vi "Resize Value Columns.vi"(8 "error in":errorcluster, 9 "Item Names":string[][](array[string]), 10 "Column Header":string[](array[string]), 11 "Report Viewer in":refnum<class "Report Viewer.lvclass">) -> (0 "error out":errorcluster, 3 "Report Viewer out":refnum<class "Report Viewer.lvclass">)   [LabVIEW 2023, in "Report Viewer.lvlib" / "Report Viewer.lvclass"]
uses:
  Library/Report Viewer.lvclass
  Library/Report Viewer.lvclass/Report Viewer.ctl
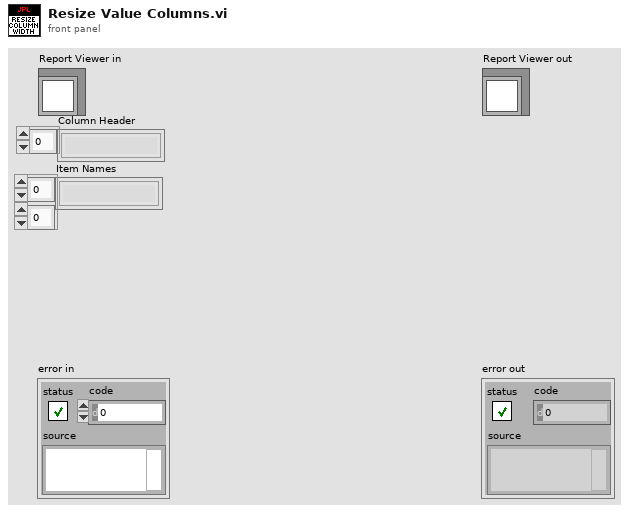
[diagram p1: front panel]
types:
  T1 = enum16{"User-specified Font", "Application Font", "System Font", "Dialog Font"}
  T2 = cluster{"left":i16, "top":i16, "right":i16, "bottom":i16}
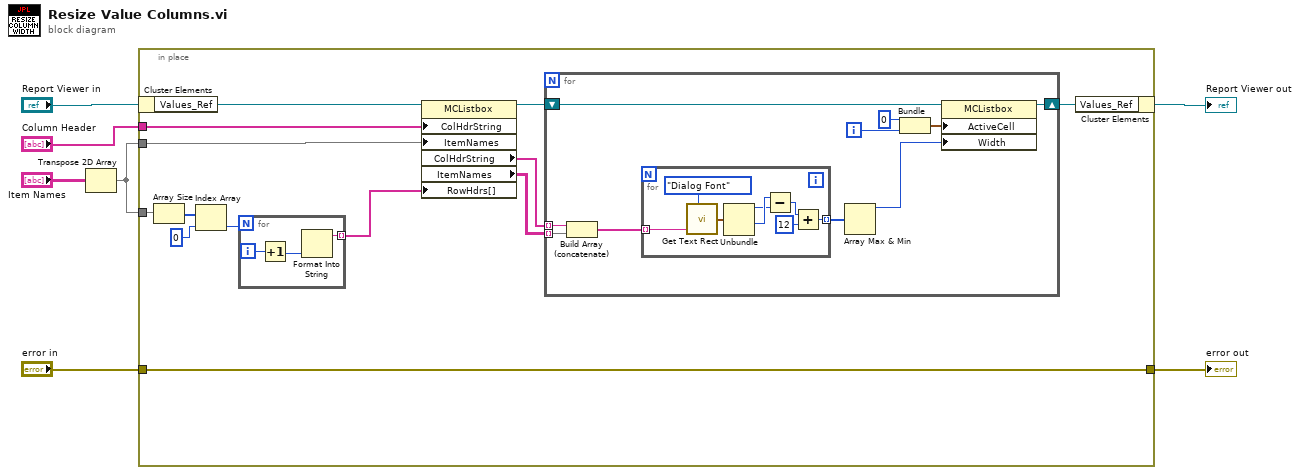
[diagram p0: block diagram]
diagram:
  n1 = Transpose 2D Array(2D array="Item Names") -> (transposed array=w1:string[][])
  n2 = in-place {
    in-place-border: "error in" -> [w15]
    in-place-border: [w15] -> w4
    in-place-border: "Column Header" -> [w14]
    in-place-border: w1 -> [w13]
    in-place-border: w1 -> [w12]
    n3 = in-place-cluster #1("Report Viewer in") -> ("Values_Ref"=w20:refnum<vi>)
    n4 = Array Size(array=w12) -> (size(s)=w11:i32[])
    n5 = Index Array(array=w11, index=0) -> (element=w9:i32)
    n6 = for {
      N: w9 -> [_]
      tunnel: [w21] -> w8 mode=indexing
      i -> [w23]
      n7 = Increment(x=w23) -> (x+1=w22:i32)
      n8 = Format Into String(w22) -> (resulting string=w21:string)  [unwired: 3 in, 1 out]
    }
    n9 = property class="MCListbox"(reference=w20, "ColHdrString"=w14, "ItemNames"=w13, "RowHdrs[]"=w8) -> (reference out=w19:refnum<vi>, "ColHdrString"=w18:string[], "ItemNames"=w17:string[][])  [unwired: 1 in, 1 out]
    n10 = for {
      tunnel: w17 -> [w27] mode=indexing
      tunnel: w18 -> [w28] mode=indexing
      shift-right: [w25] -> w16
      shift-left: w19 -> [w29]
      i -> [w24]
      n11 = Build Array (concatenate)(w28, w27) -> (w26:string[])
      n12 = for {
        tunnel: [w36] -> w32 mode=indexing
        tunnel: w26 -> [w34] mode=indexing
        n13 = call <vilib>:"Get Text Rect.vi"("desired font(Application)"=T1."Dialog Font", "text"=w34) -> ("rect"=w41:T2)  [unwired: 7 in]
        n14 = Unbundle(w41) -> ("left"=w39:i16, "right"=w40:i16)  [unwired: 2 out]
        n15 = Subtract(x=w40, y=w39) -> (x-y=w38:i16)
        n16 = Add(x=w38, y=i16 12) -> (x+y=w36:i16)
      }
      n17 = Array Max & Min(array=w32) -> (max value=w31:i16)  [unwired: 3 out]
      n18 = Bundle(0, w24) -> (w33:cluster{i32, i32})  [unwired: 1 in]
      n19 = property on="Property Node" class="MCListbox"(reference=w29, "ActiveCell"=w33, "Width"=w31) -> (reference out=w25:refnum<vi>)  [unwired: 1 in, 1 out]
    }
    n20 = in-place-cluster #1("Values_Ref"=w16) -> (→"Report Viewer out":refnum<class "Report Viewer.lvclass">)
  }
  "error out" <- w4
